vi "MessageQueue_EnqueueElement.vi"(0 "QueueIn":refnum<queue>, 2 "Message":string, 3 "Data":variant, 5 "ErrorIn":errorcluster, 9 "HighPriority":bool) -> (14 "QueueOut":refnum<queue>, 19 "ErrorOut":errorcluster)   [LabVIEW 2016]
doc: "Schiebt ein Element in die Queue. Mit HighPriority wird das Element auf der anderen Seite hineingelegt, wo es als erstes wieder abgearbeitet werden kann\n\nsige / 4.12.13"
uses:
  private/MessageQueue.MessageTypeDef.ctl
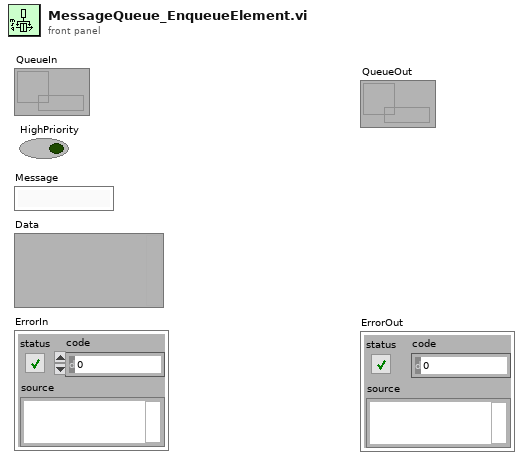
[diagram p1: front panel]
types:
  T1 = typedef "MessageQueue.MessageTypeDef.ctl" = cluster{"Message":string, "Data":variant}
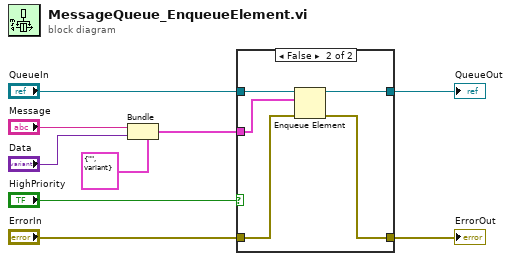
[diagram p0: block diagram]
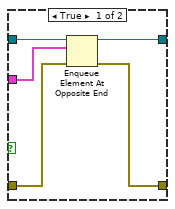
[diagram p2: hidden frame]
diagram:
  n1 = Bundle(cluster=T1 {"Message"="", "Data"=variant} ("Cluster"), "Message"="Message", "Data"="Data") -> (w4:T1)
  n2 = case shown="False" "HighPriority" {
    tunnel: "QueueIn" -> [w14 w19]
    tunnel: "ErrorIn" -> [w13 w18]
    tunnel: [w12 w17] -> w7
    tunnel: [w11 w16] -> w6
    tunnel: w4 -> [w10 w15]
    frame True {
      n3 = Enqueue Element At Opposite End(queue=w14, element=w10, error in (no error)=w13) -> (queue out=w11:refnum<queue>, error out=w12:errorcluster)  [unwired: 1 in, 1 out]
    }
    frame False {
      n4 = Enqueue Element(queue=w19, element=w15, error in (no error)=w18) -> (queue out=w16:refnum<queue>, error out=w17:errorcluster)  [unwired: 1 in, 1 out]
    }
  }
  "ErrorOut" <- w7
  "QueueOut" <- w6
